vi "Time String(us).vi"() -> (2 "system time string(us)":string)   [LabVIEW 2020]
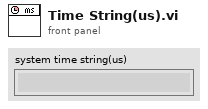
[diagram p1: front panel]
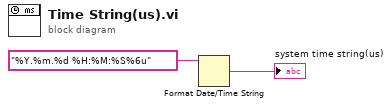
[diagram p0: block diagram]
diagram:
  n1 = Format Date/Time String(time format string (%c)="%Y.%m.%d %H:%M:%S%6u") -> (date/time string=→"system time string(us)":string)  [unwired: 2 in]
